vi "Thread.vi"(8 "error in (no error)":errorcluster, 11 "Singleton in":refnum<class "Singleton.lvclass">) -> (0 "error out":errorcluster)   [LabVIEW 2014, in "Singleton.lvlib" / "Singleton.lvclass"]
uses:
  Singleton.lvclass
  Singleton.lvclass/Singleton.ctl
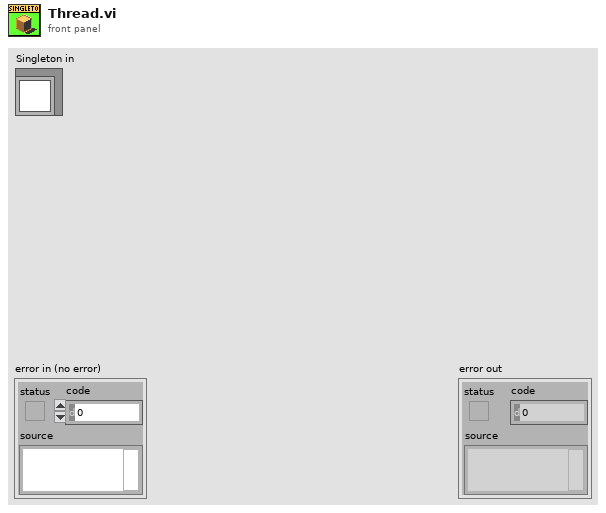
[diagram p1: front panel]
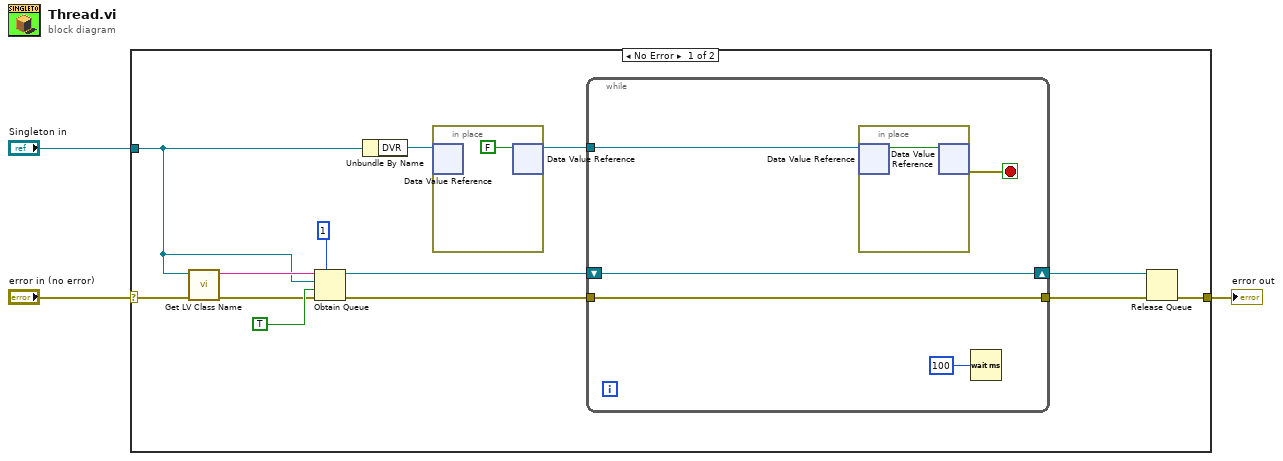
[diagram p0: block diagram]
diagram:
  n1 = case shown="No Error" "error in (no error)" {
    selector: "error in (no error)" -> [w8 w24]
    tunnel: [w7 w24] -> w2
    tunnel: "Singleton in" -> [w5 _]
    frame No Error {
      n2 = call <vilib>:"Get LV Class Name.vi"("error in (no error)"=w8, "object"=w5) -> ("error out"=w13:errorcluster, "class name"=w16:string)  [unwired: 8 in]
      n3 = Obtain Queue(max queue size (-1, unlimited)=1, name (unnamed)=w16, element data type=w5, create if not found? (T)=TRUE, error in (no error)=w13) -> (queue out=w12:refnum<queue>, error out=w11:errorcluster)  [unwired: 1 out]
      n4 = Unbundle By Name(w5) -> ("DVR"=w6:refnum<data-value>)
      n5 = in-place {
        n6 = in-place-dvr #1(w6) -> ()  [unwired: 2 out]
        n7 = in-place-dvr #1(FALSE ("data value")) -> (w4:refnum<data-value>)  [unwired: 1 out]
      }
      n8 = while {
        shift-right: [w22] -> w10
        shift-left: w12 -> [w22]
        tunnel: w11 -> [w21]
        tunnel: [w21] -> w9
        tunnel: w4 -> [w20]
        stop <- w18 stop-if-true
        n9 = in-place {
          n10 = in-place-dvr #2(w20) -> (w23:bool)  [unwired: 1 out]
          n11 = in-place-dvr #2(w23) -> (w18:errorcluster)  [unwired: 1 out]
        }
        n12 = Wait (ms)(milliseconds to wait=u32 100) -> ()  [unwired: 1 out]
      }
      n13 = Release Queue(queue=w10, error in (no error)=w9) -> (error out=w7:errorcluster)  [unwired: 1 in, 2 out]
    }
    frame Error {
    }
  }
  "error out" <- w2
